vi "Timing Process.vi"(0 "Initial States":u16[](array[numeric]), 1 "Switching Times":u32[][](array[numeric]), 2 "Total Steps":u64, 3 "error in (no error)":errorcluster, 4 "Channel":u16) -> (5 "Output Signal Array":i16[][](array[numeric]) format="%b", 6 "Output Time Array":i32[](array[numeric]), 7 "error out":errorcluster)   [LabVIEW 2012]
panel:
  # "This Programs Translates Timing File into Output Signal Array (2D) and Output Time Stamp Array (1D)"
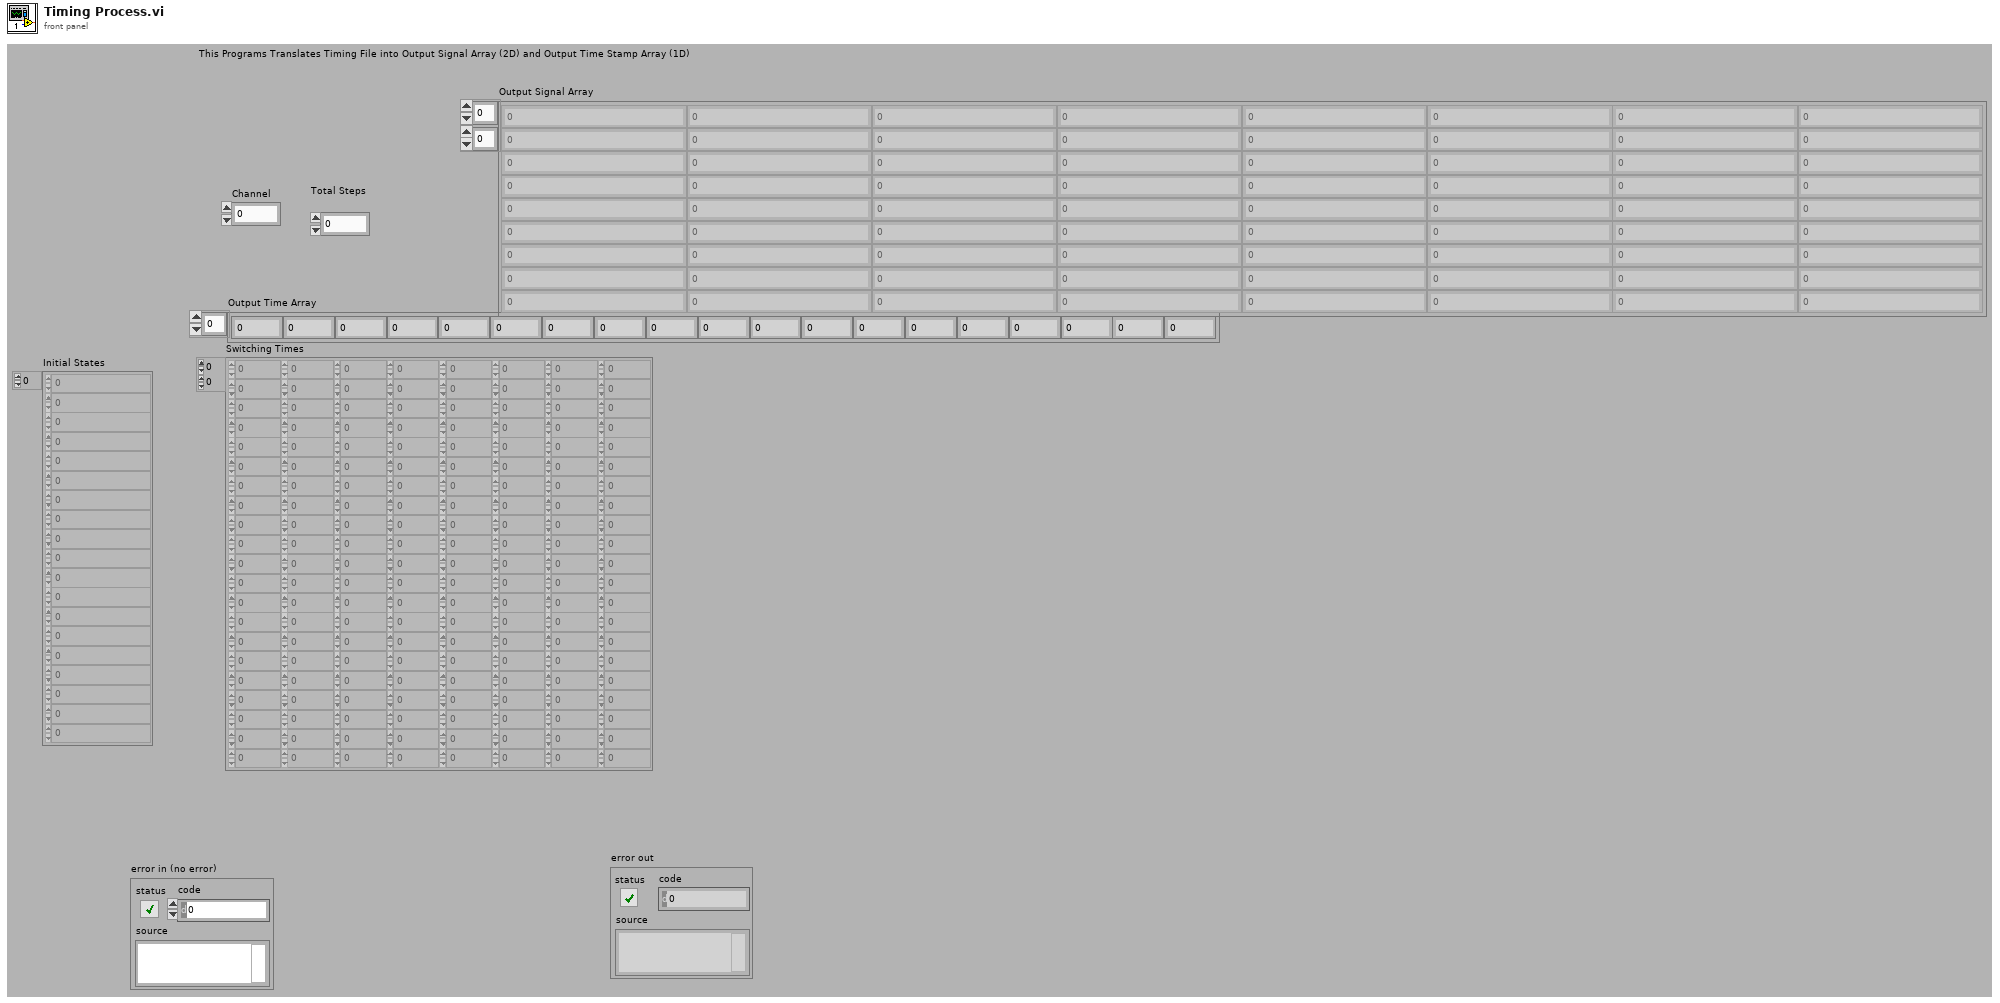
[diagram p1: front panel]
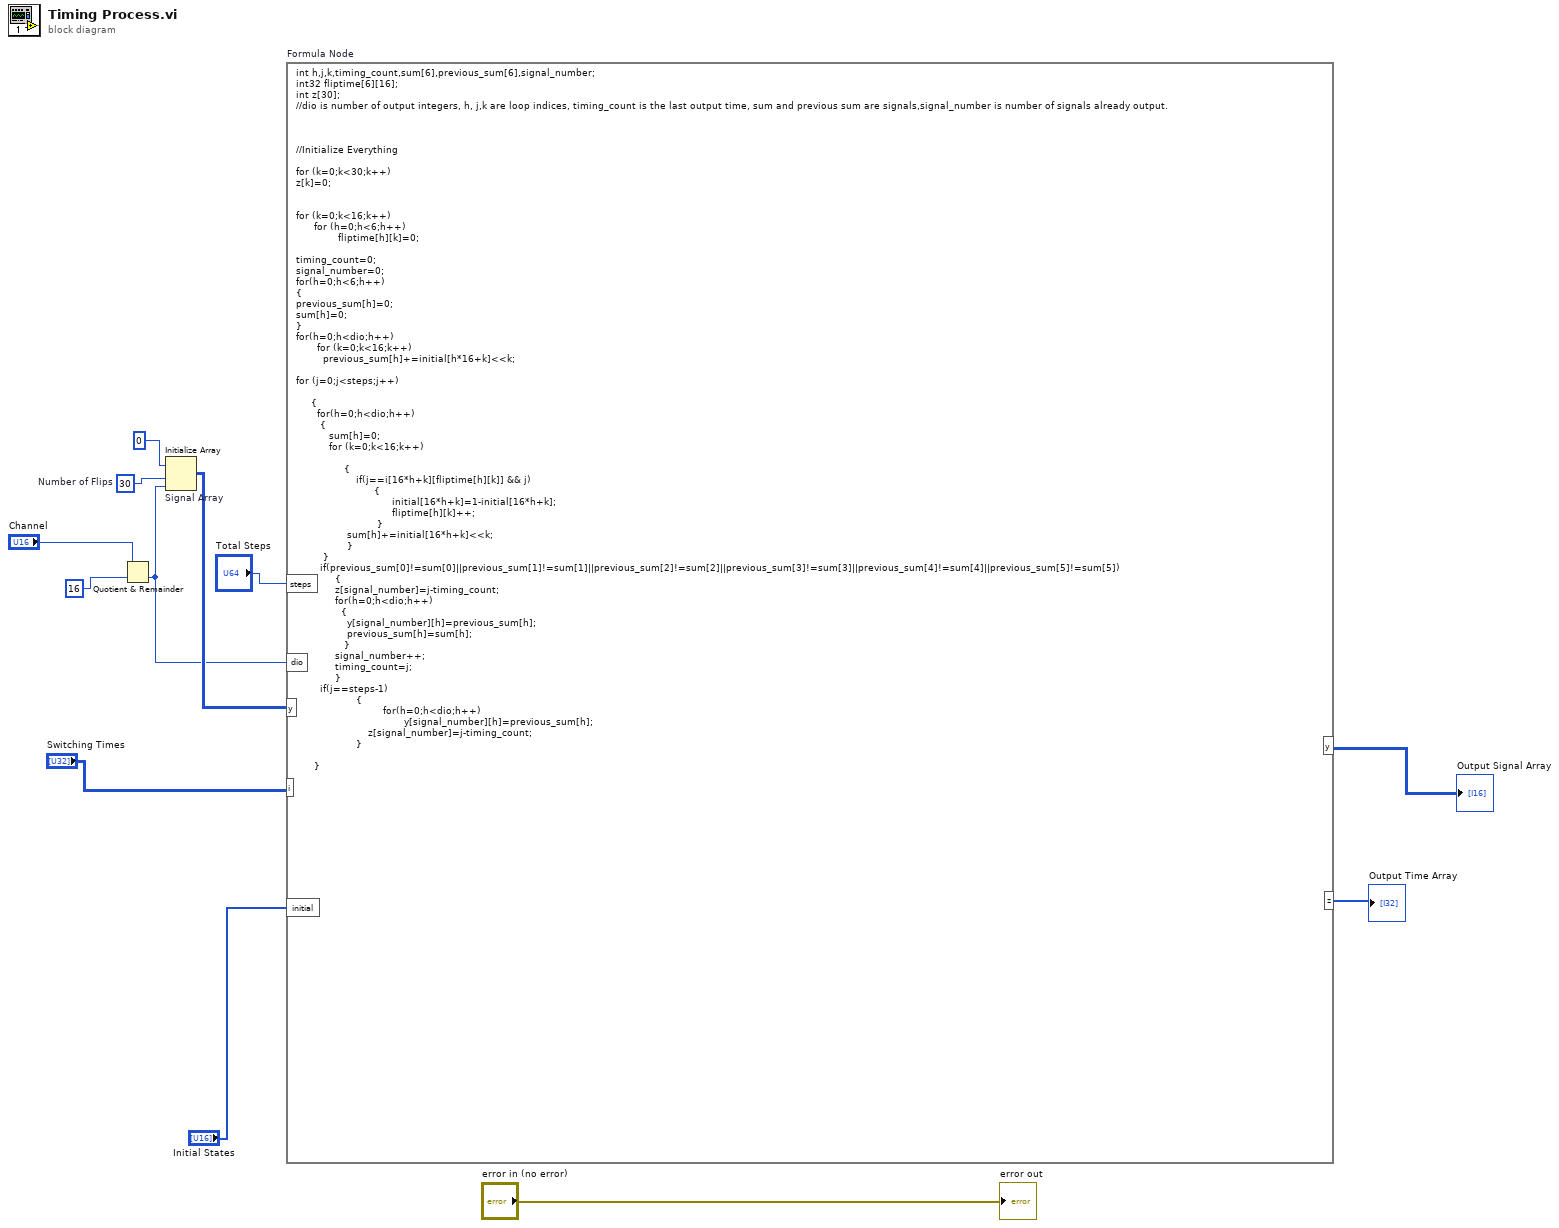
[diagram p0: block diagram]
diagram:
  w7 = 30  # Number of Flips
  n1 = Quotient & Remainder(x="Channel", y=u16 16) -> (floor(x/y)=w3:u16)  [unwired: 1 out]
  n2 = Initialize Array "Signal Array"(u16 0, w7, w3) -> (w4:u16[][])
  n3 = formula code="int h,j,k,timing_count,sum[6],previous_sum[6],signal_number;\nint32 fliptime[6][16];\nint z[30];\n//dio is number of output integers, h, j,k are loop indices, timing_count is the last output time, sum and previous sum are signals,signal_number is number of signals already output.\n\n\n\n//Initialize Everything\n\nfor (k=0;k<30;k++)\nz[k]=0;\n\n\nfor (k=0;k<16;k++)\n      for (h=0;h<6;h++)\n              fliptime[h][k]=0;\n\ntiming_count=0;\nsignal_number=0;\nfor(h=0;h<6;h++)\n{\nprevious_sum[h]=0;\nsum[h]=0;\n}\nfor(h=0;h<dio;h++)\n       for (k=0;k<16;k++)\n         previous_sum[h]+=initial[h*16+k]<<k;\n\nfor (j=0;j<steps;j++) \n\n     {\n       for(h=0;h<dio;h++)\n        {\n           sum[h]=0;\n           for (k=0;k<16;k++)\n\n                {\n                    if(j==i[16*h+k][fliptime[h][k]] && j)\n                          {\n                                initial[16*h+k]=1-initial[16*h+k];\n                                fliptime[h][k]++;\n                           }\n                 sum[h]+=initial[16*h+k]<<k;\n                 }\n         }\n        if(previous_sum[0]!=sum[0]||previous_sum[1]!=sum[1]||previous_sum[2]!=sum[2]||previous_sum[3]!=sum[3]||previous_sum[4]!=sum[4]||previous_sum[5]!=sum[5])\n             {        \n             z[signal_number]=j-timing_count;\n             for(h=0;h<dio;h++)\n               {\n                 y[signal_number][h]=previous_sum[h];       \n                 previous_sum[h]=sum[h];\n                }\n             signal_number++;\n             timing_count=j;\n             }\n        if(j==steps-1)\n                    { \n                             for(h=0;h<dio;h++)\n                                    y[signal_number][h]=previous_sum[h];\n                        z[signal_number]=j-timing_count;\n                    }\n          \n      }"("i"="Switching Times", "initial"="Initial States", "steps"="Total Steps", "dio"=w3, "y"=w4) -> ("y"=→"Output Signal Array":u16[][], "z"=→"Output Time Array":i32[])
  "error out" <- "error in (no error)"
